vi "Signal Stop Event.vi"   [LabVIEW 2013]
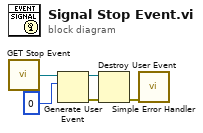
[diagram p0: block diagram]
diagram:
  n1 = call "GET Stop Event.vi"() -> ("Stop Event"=w5:refnum<user-event>)
  n2 = Generate User Event(user event=w5, event data cluster=0 ("event data")) -> (user event out=w3:refnum<user-event>, error out=w2:errorcluster)  [unwired: 2 in]
  n3 = Destroy User Event(user event=w3, error in=w2) -> (error out=w1:errorcluster)
  n4 = call <vilib>:"Simple Error Handler.vi"("error in (no error)"=w1) -> ()  [unwired: 4 in, 5 out]
